vi "measure_internal_resistance.vi"(8 "Internal resistance parameters":T1, 11 "Array":waveform(dbl)[](array[waveform])) -> (0 "reset switch":bool, 3 "Resistenza\ninterna":dbl)   [LabVIEW 2023]
uses:
  <vilib>/Analysis/NI_AALPro.lvlib
  internal_resistance_params.ctl
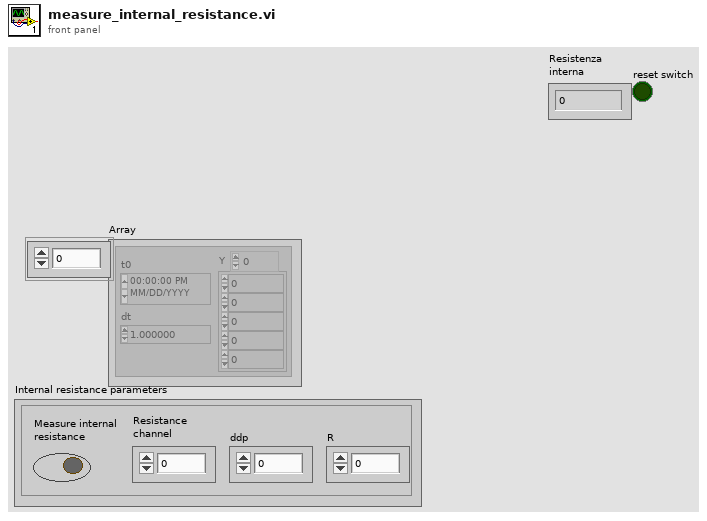
[diagram p1: front panel]
types:
  T1 = typedef "internal_resistance_params.ctl" = cluster{"Measure internal\nresistance":bool, "Resistance\nchannel":i32, "ddp":dbl, "R":dbl}
  T2 = cluster{"slope min":dbl, "slope max":dbl, "intercept min":dbl, "intercept max":dbl}
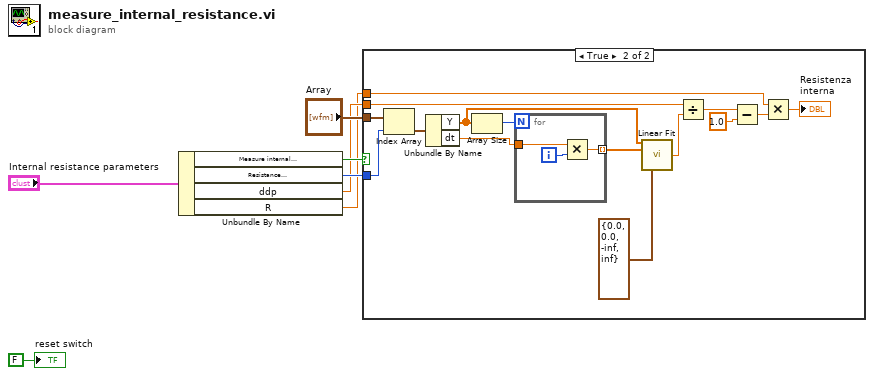
[diagram p0: block diagram]
diagram:
  n1 = Unbundle By Name("Internal resistance parameters") -> ("Measure internal\nresistance"=w4:bool, "Resistance\nchannel"=w3:i32, "ddp"=w2:dbl, "R"=w1:dbl)
  n2 = case shown="True" w4 {
    tunnel: "Array" -> [_ w12]
    tunnel: w3 -> [_ w10]
    tunnel: w2 -> [_ w9]
    tunnel: w1 -> [_ w8]
    frame False {
    }
    frame True {
      n3 = Index Array(array=w12, index=w10) -> (element=w22:waveform(dbl))
      n4 = Unbundle By Name(w22) -> ("Y"=w21:dbl[], "dt"=w19:dbl)
      n5 = Array Size(array=w21) -> (size(s)=w20:i32)
      n6 = for {
        N: w20 -> [_]
        tunnel: w19 -> [w25]
        tunnel: [w23] -> w18 mode=indexing
        i -> [w24]
        n7 = Multiply(x=w25, y=w24) -> (x*y=w23:dbl)
      }
      n8 = call <vilib>:"Linear Fit.vi"("Y"=w21, "X"=w18, "parameter bounds"=T2 {"slope min"=0.0, "slope max"=0.0, "intercept min"=-inf, "intercept max"=inf}) -> ("intercept"=w13:dbl)  [unwired: 8 in, 4 out]
      n9 = Divide(x=w9, y=w13) -> (x/y=w15:dbl)
      n10 = Subtract(x=w15, y=1.0) -> (x-y=w16:dbl)
      n11 = Multiply(x=w8, y=w16) -> (x*y=→"Resistenza\ninterna":dbl)
    }
  }
  "reset switch" <- FALSE ("Measure internal\nresistance")
